vi "Read Status.vi"(11 "Test Case Result In":refnum<class "Test Case Result.lvclass">) -> (1 "Glyph Index":i32, 2 "Status":T1, 3 "Test Case Result Out":refnum<class "Test Case Result.lvclass">)   [LabVIEW 2020, in "Test Case Result.lvclass"]
uses:
  Test Case Result.lvclass
  Assertion Result/Public/TypeDefs/Status.ctl
  Test Case Result.lvclass/Test Case Result.ctl
  Method Result/Method Result.lvclass/Method Result.ctl
  Assertion Result/Assertion Result.lvclass
  Method Result/Method Result.lvclass
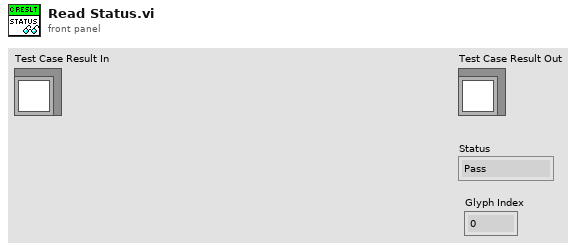
[diagram p1: front panel]
types:
  T1 = typedef "Assertion Result.lvclass/Status.ctl" = enum16{"Pass", "Fail", "Error", "Skipped", "Setup Error", "Broken", "Teardown Error"}
  T2 = map{string, refnum<class "Method Result.lvclass">}
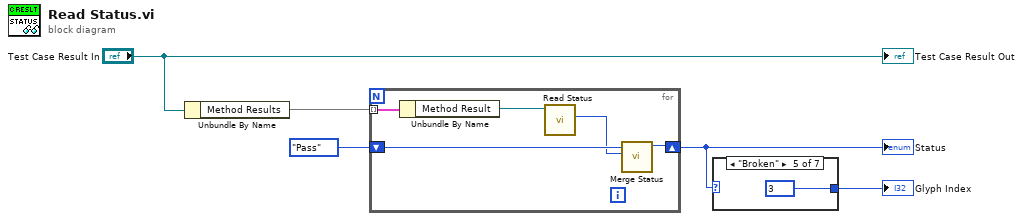
[diagram p0: block diagram]
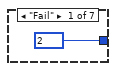
[diagram p2: hidden frame]
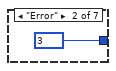
[diagram p3: hidden frame]
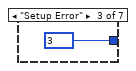
[diagram p4: hidden frame]
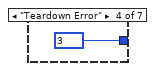
[diagram p5: hidden frame]
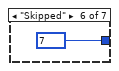
[diagram p6: hidden frame]
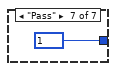
[diagram p7: hidden frame]
diagram:
  n1 = Unbundle By Name("Test Case Result In") -> ("Method Results"=w2:T2)
  n2 = for {
    shift-right: [w8] -> w1
    shift-left: Status."Pass" ("Status") -> [w10]
    tunnel: w2 -> [w6] mode=indexing
    n3 = Unbundle By Name(w6) -> ("Method Result"=w7:refnum<class "Method Result.lvclass">)
    n4 = call "Read Status.vi"("Method Result In"=w7) -> ("Status"=w9:T1)  [unwired: 8 in, 2 out]
    n5 = call "Merge Status.vi"("New"=w9, "Current"=w10) -> ("Merged"=w8:T1)  [unwired: 9 in]
  }
  "Status" <- w1
  n6 = case shown="\"Broken\"" w1 {
    tunnel: [2 ("Listbox Symbol Ring Constant") 3 ("Listbox Symbol Ring Constant") 3 ("Listbox Symbol Ring Constant") 3 ("Listbox Symbol Ring Constant") 3 ("Listbox Symbol Ring Constant") 7 ("Listbox Symbol Ring Constant") 1 ("Listbox Symbol Ring Constant")] -> w4
    frame "Fail" {
    }
    frame "Error" {
    }
    frame "Setup Error" {
    }
    frame "Teardown Error" {
    }
    frame "Broken" {
    }
    frame "Skipped" {
    }
    frame "Pass" {
    }
  }
  "Glyph Index" <- w4
  "Test Case Result Out" <- "Test Case Result In"
